vi "Close Online Input.vi"(8 "Error In":errorcluster, 11 "Config In":T2 {"task ID" format="%.0x"}) -> (0 "Error Out":errorcluster)   [LabVIEW 2014, in "Aquisicao de Dados.lvlib"]
uses:
  <vilib>/sound2/lvsound2.llb/Sound Input Task ID.ctl
  Aquisicao de Dados.lvlib
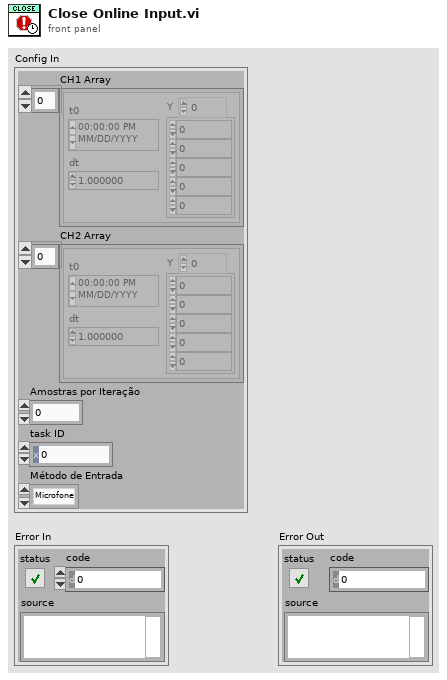
[diagram p1: front panel]
types:
  T1 = typedef "Sound Input Task ID.ctl" = u32
  T2 = cluster{"CH1 Array":waveform(dbl)[], "CH2 Array":waveform(dbl)[], "Amostras por Iteração":i32, "task ID":T1, "Método de Entrada":enum16{"Microfone", "Arduino", "LTSpice", "Arquivo WAV"}}
  T3 = enum16{"Microfone", "Arduino", "LTSpice", "Arquivo WAV"}
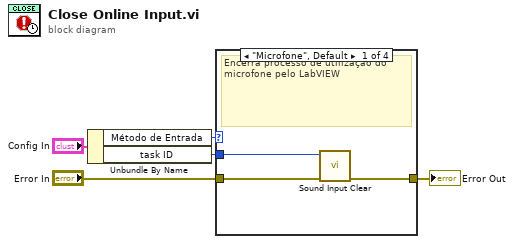
[diagram p0: block diagram]
diagram:
  n1 = Unbundle By Name("Config In") -> ("Método de Entrada"=w4:T3, "task ID"=w5:T1)
  n2 = case shown="\"Microfone\", Default" w4 {
    tunnel: [w8 w9 w10 w11] -> w1
    tunnel: "Error In" -> [w7 w9 w10 w11]
    tunnel: w5 -> [w6 _ _ _]
    frame "Microfone", Default {
      # "Encerra processo de utilização do microfone pelo LabVIEW"
      n3 = call <vilib>:"Sound Input Clear.vi"("error in (no error)"=w7, "task ID"=w6) -> ("error out"=w8:errorcluster)  [unwired: 9 in]
    }
    frame "Arduino" {
    }
    frame "LTSpice" {
    }
    frame "Arquivo WAV" {
    }
  }
  "Error Out" <- w1
